vi "example_GArrayDownloadFile.vi"() -> ()   [LabVIEW 2021]
uses:
  <vilib>/Galil/resources/gclib32/gclib32.lvlib
  <vilib>/Galil/resources/gclibo32/gclibo32.lvlib
panel:
  in  "File Location":string="C:\\Program Files (x86)\\Galil\\gclib\\examples\\labview\\array_download.csv"
  out "Error Out":errorcluster
  in  "IP Address":string="192.168.1.77"
  out "Response":string
  in  "Command":string="LA"
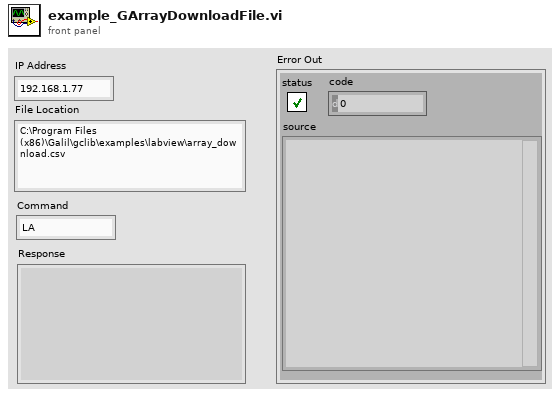
[diagram p1: front panel]
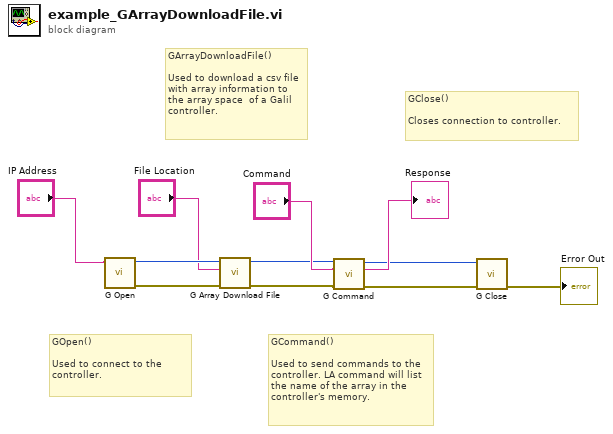
[diagram p0: block diagram]
diagram:
  # "GClose()\n\nCloses connection to controller."
  # "GCommand()\n\nUsed to send commands to the controller. LA command will list the name of the array in the controller's memory."
  # "GArrayDownloadFile()\n\nUsed to download a csv file with array information to the array space  of a Galil controller."
  # "GOpen()\n\nUsed to connect to the controller."
  n1 = call <vilib>:"G Open.vi"("address"="IP Address") -> ("error out"=w3:errorcluster, "g out"=w5:u32)  [unwired: 8 in]
  n2 = call <vilib>:"G Array Download File.vi"("error in (no error)"=w3, "file_path"="File Location", "g"=w5) -> ("error out"=w2:errorcluster, "g out"=w1:u32)  [unwired: 7 in]
  n3 = call <vilib>:"G Command.vi"("g"=w1, "command"="Command", "error in (no error)"=w2) -> ("g out"=w7:u32, "buffer out"=→"Response":string, "error out"=w6:errorcluster)  [unwired: 10 in]
  n4 = call <vilib>:"G Close.vi"("error in (no error)"=w6, "g"=w7) -> ("error out"=→"Error Out":errorcluster)  [unwired: 9 in]
